vi "Read lockin vs time_1.0.vi"(8 "stop":bool, 10 "Comments":string="SA02610M 20130128\ncool down\n", 11 "folder name":string="monitor lockin") -> (1 "X1":cluster{"Y":dbl[], "Y":dbl[]}[](graph), 3 "Temp vs Time":cluster{"Y":dbl[], "Y":dbl[]}[](graph), 5 "X4":cluster{"Y":dbl[], "Y":dbl[]}[](graph))   [LabVIEW 2013]
uses:
  <userlib>/Levylab/PPMS VI/Lock-in Globles.vi
  <userlib>/Levylab/PPMS VI/SubVI/ITX_Global.vi
  cryogenic ltd/state machine/state machine/Cryogeni Global 1.vi
  <vilib>/Utility/file.llb/Write To Spreadsheet File (string).vi
panel:
  in  "Tab Control":T1(tab)
  in  "milliseconds to wait":u32=1000
  out "Connected":string="I-:4\nV2+:28\nI+:1\nV1+:2\nV-:3\nV2-:5\n"
  in  "Lockins":i32[](array[numeric])=[0, 1, 2, 3, 4, 5]
  out "Array X":dbl[](array[numeric])
  out "Array Y":dbl[](array[numeric])
  out "X0":cluster{"Y":dbl[], "Y":dbl[]}[](graph)
  out "X2":cluster{"Y":dbl[], "Y":dbl[]}[](graph)
  out "X3":cluster{"Y":dbl[], "Y":dbl[]}[](graph)
  out "X5":cluster{"Y":dbl[], "Y":dbl[]}[](graph)
  out "R":cluster{"Y":dbl[], "Y":dbl[]}[](graph)
  in  "V1":i32
  in  "Current":i32
  in  "V2":i32
  out "B vs Time":cluster{"Y":dbl[], "Y":dbl[]}[](graph)
  out "R vs T":cluster{"Y":dbl[], "Y":dbl[]}[](graph)
  # "0,1,2,3 ect."
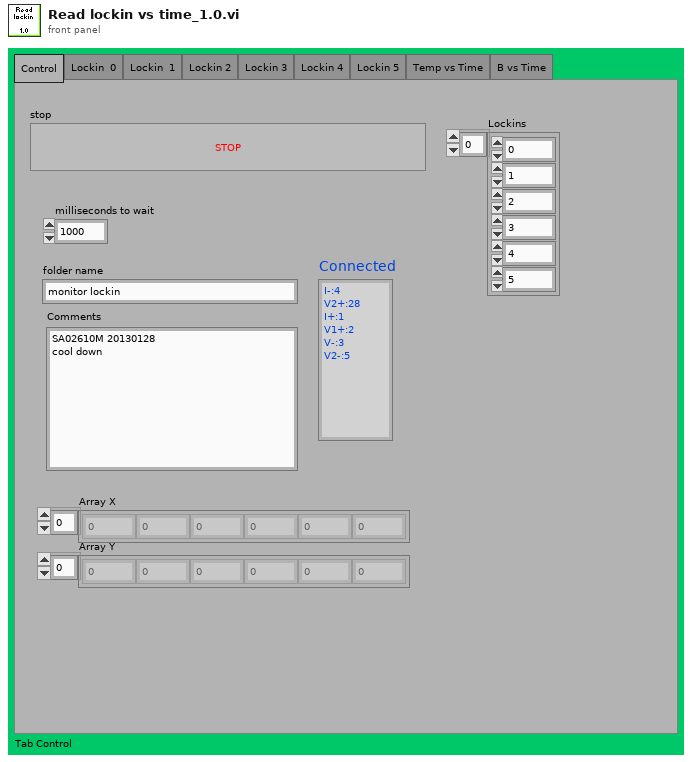
[diagram p1: front panel]
types:
  T1 = enum32{"Control", "Lockin  0", "Lockin  1", "Lockin 2", "Lockin 3", "Lockin 4", "Lockin 5", "Temp vs Time", "B vs Time"}
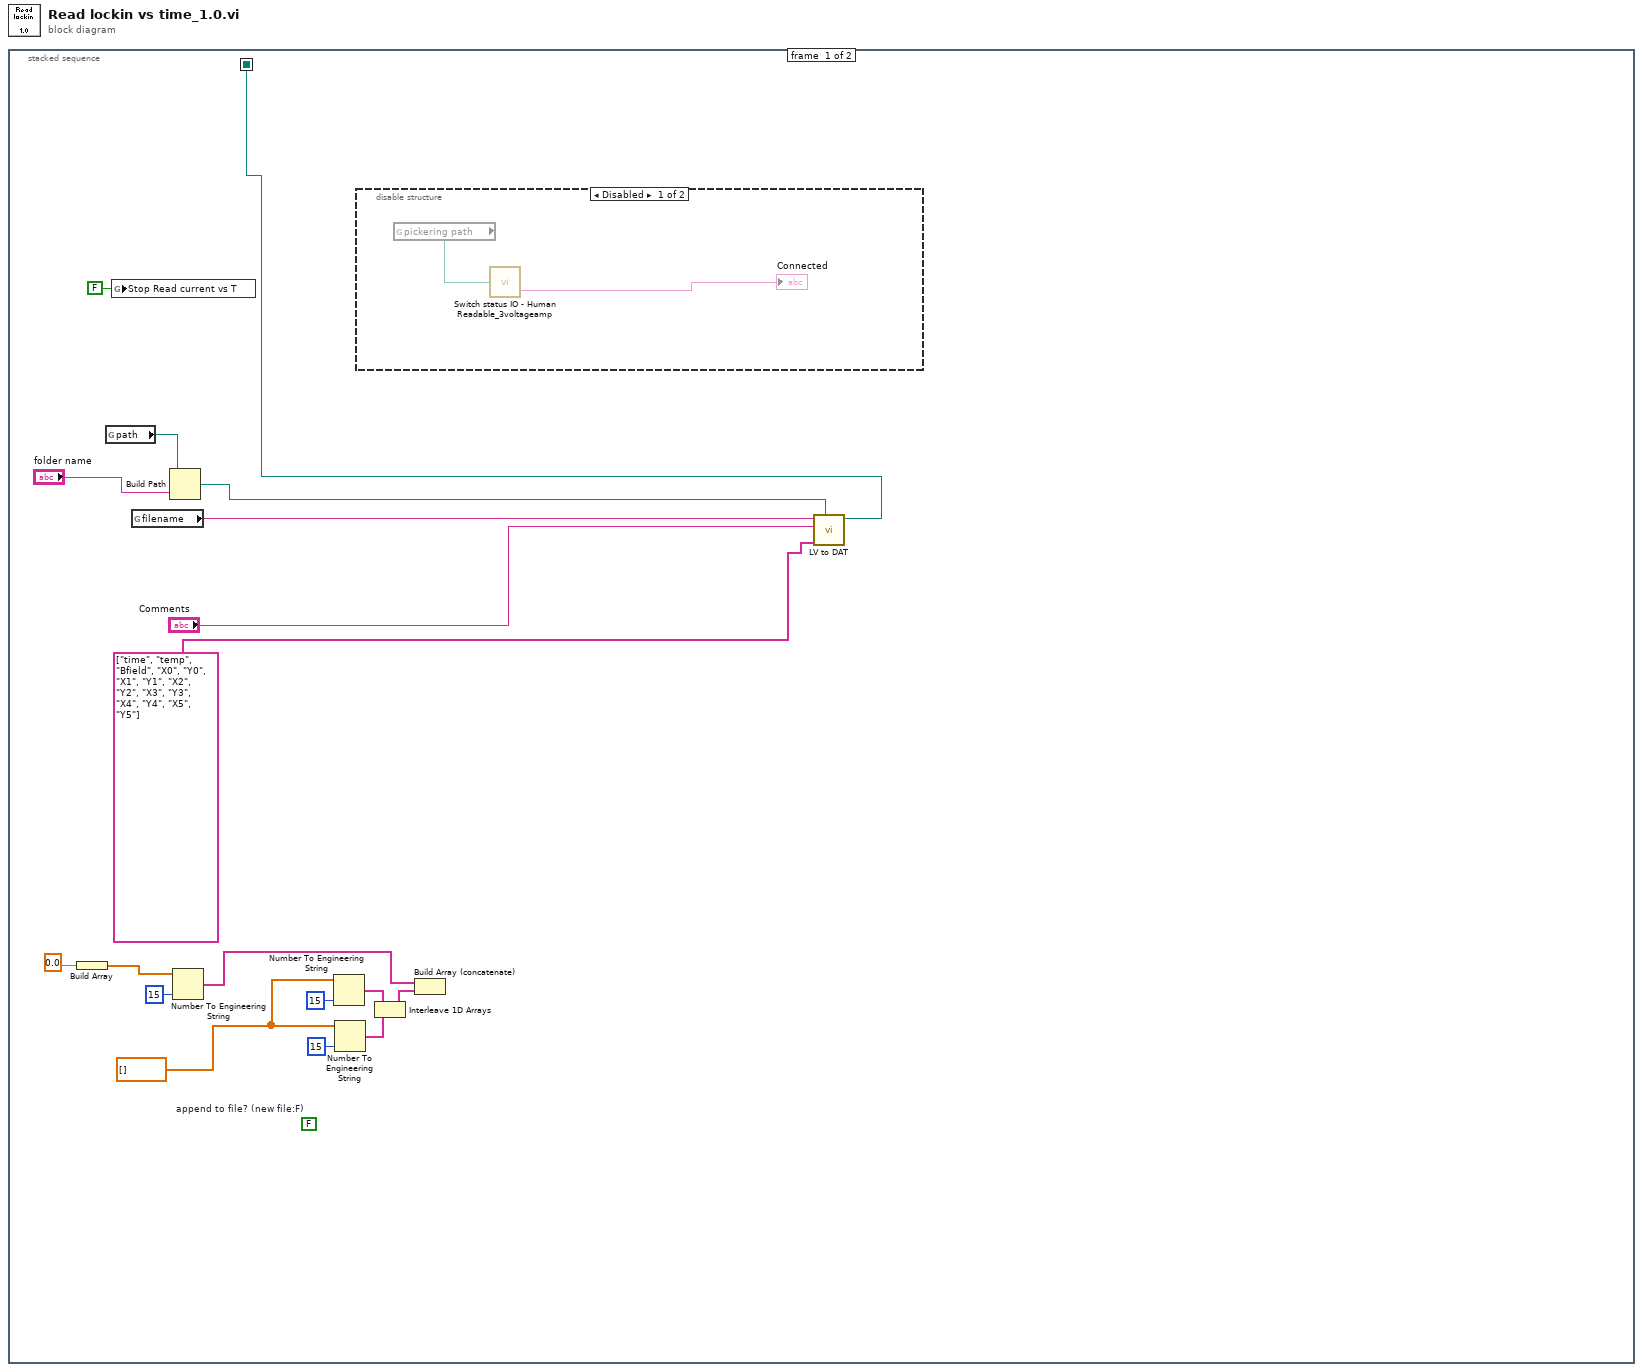
[diagram p0: block diagram]
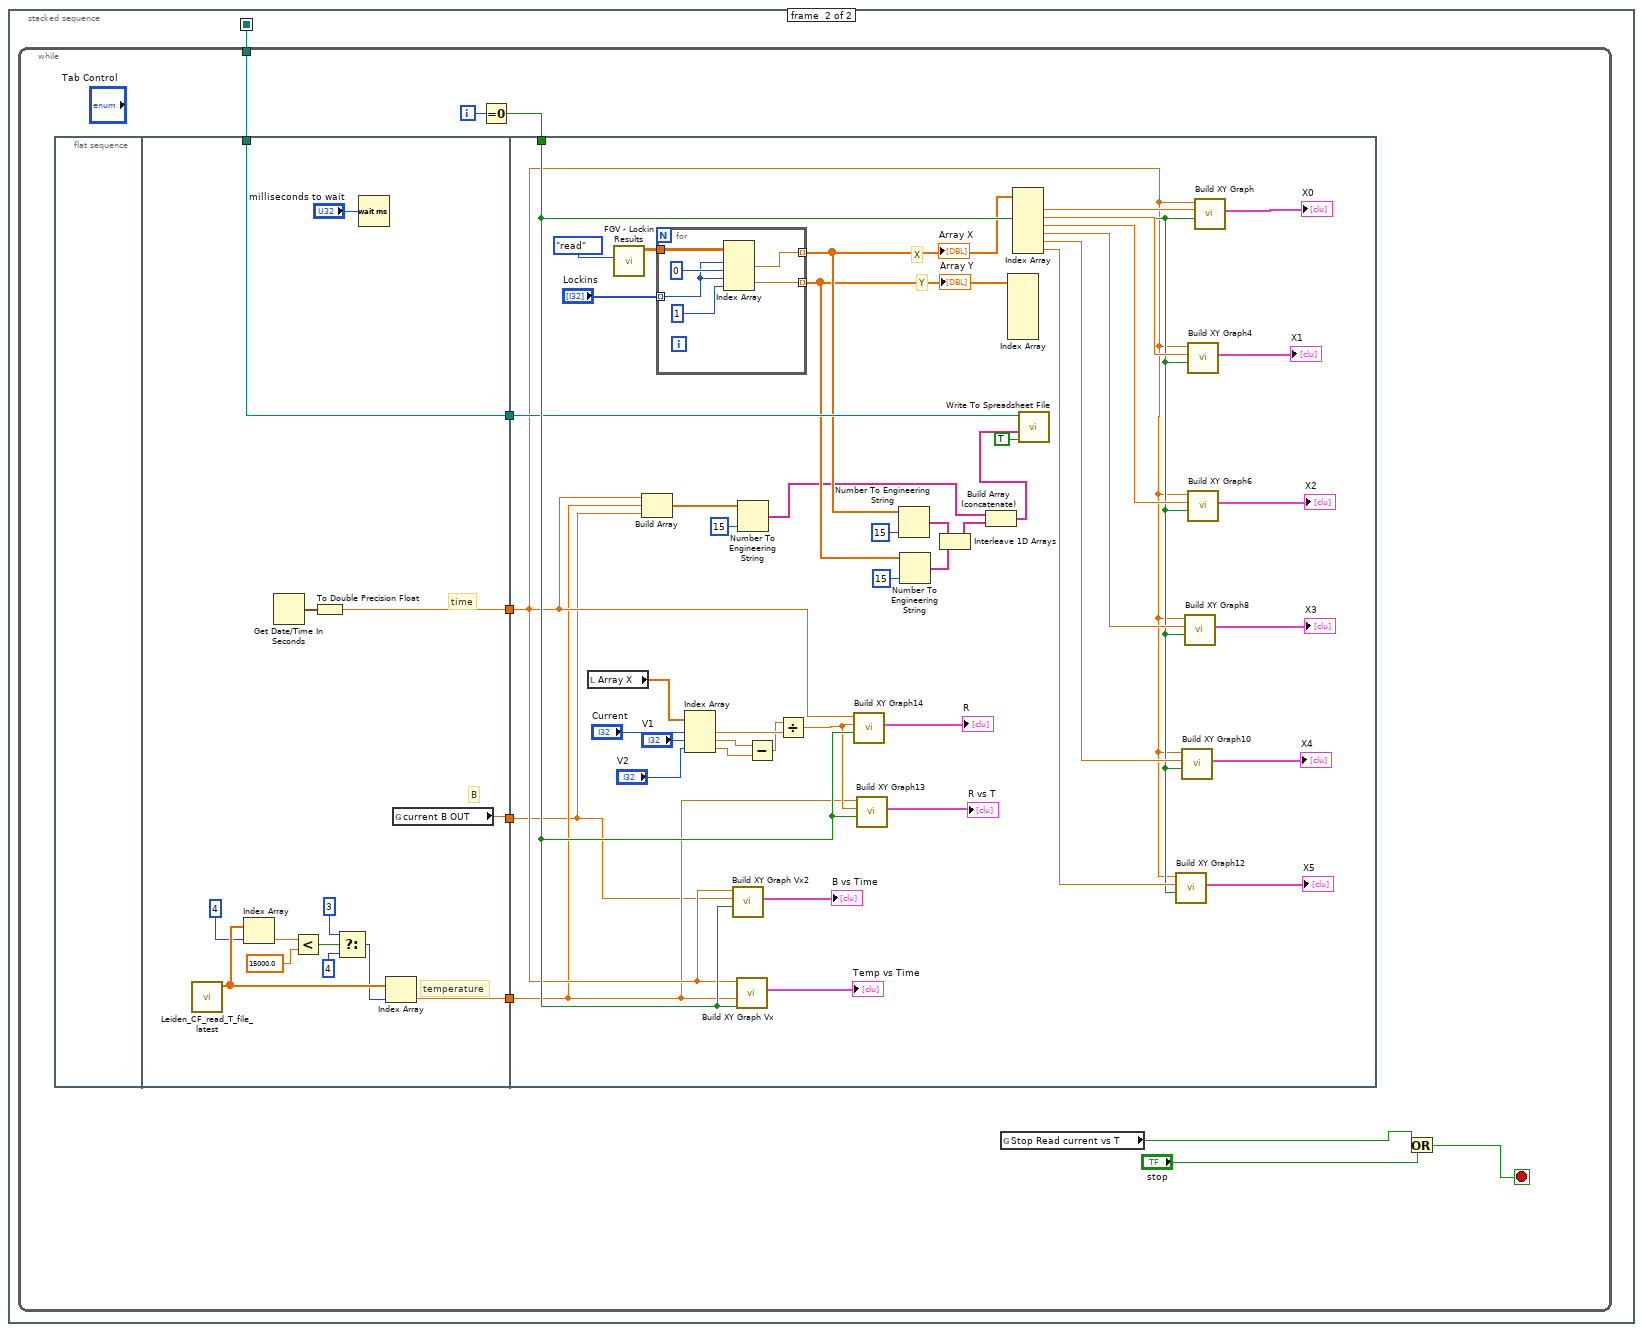
[diagram p3: hidden frame]
diagram:
  n1 = stacked-sequence {
    seq-local: [w1 _] -> [_ w23]
    frame #0 {
      w7 = dbl[] []
      w17 = FALSE  # append to file? (new file:F)
      n2 = Build Array(0.0) -> (w13:dbl[])
      n3 = global read "ITX_Global.vi" "path"() -> (w19:path)
      n4 = global write "Lock-in Globles.vi" "Stop Read current vs T"(FALSE ("Stop Read current vs T")) -> ()
      n5 = global read "ITX_Global.vi" "filename"() -> (w3:string)
      n6 = Build Path(base path=w19, name or relative path="folder name") -> (appended path=w2:path)
      n7 = Number To Engineering String(2:i16 15 ("precision (6)"), 4:w13) -> (0:w12:string[])  [unwired: 2 out]
      n8 = Number To Engineering String(2:i16 15 ("precision (6)"), 4:w7) -> (0:w11:string[])  [unwired: 2 out]
      n9 = Number To Engineering String(2:i16 15 ("precision (6)"), 4:w7) -> (0:w10:string[])  [unwired: 2 out]
      n10 = disable-structure shown="Disabled" {
        frame Disabled {
          n11 = global read "ITX_Global.vi" "pickering path"() -> (w21:path)
          n12 = call <userlib>:"Switch status IO - Human Readable_3voltageamp.vi"("Switch status"=w21) -> ("String"=→"Connected":string)  [unwired: 3 in]
        }
        frame Enabled {
        }
      }
      n13 = Interleave 1D Arrays(w11, w10) -> (w9:string[])
      n14 = Build Array (concatenate)(w12, w9) -> (w6:string[])
      n15 = call <userlib>:"LV to DAT.vi"("path"=w2, "wavenames (.Vx, etc)"=string[] ["time", "temp", "Bfield", "X0", "Y0", "X1", "Y1", "X2", "Y2", "X3", "Y3", "X4", "Y4", "X5", "Y5"], "Comments"="Comments", "filename"=w3) -> ("new file path (Not A Path if cancelled)"=w1:path)  [unwired: 7 in]
    }
    frame #1 {
      n16 = while {
        tunnel: w23 -> [w26]
        i -> [w33]
        stop <- w27 stop-if-true
        n17 = flat-sequence {
          tunnel: [w45] -> w31
          tunnel: [w44] -> w29
          tunnel: [w43] -> w28
          tunnel: w26 -> [w35]
          tunnel: [w35] -> w25
          tunnel: w32 -> [w69]
          tunnel: w31 -> [w57]
          tunnel: w29 -> [w56]
          tunnel: w28 -> [w55]
          tunnel: w25 -> [w67]
          frame #0 {
          }
          frame #1 {
            # "B"
            # "time"
            # "temperature"
            n18 = call "Leiden_CF_read_T_file_latest.vi"() -> ("T array"=w42:dbl[])  [unwired: 11 in]
            n19 = Index Array(array=w42, index=4) -> (element=w40:dbl)
            n20 = Get Date/Time In Seconds() -> (seconds since 1Jan1904=w46:timestamp)
            n21 = Less?(x=w40, y=15000.0) -> (x < y?=w38:bool)
            n22 = To Double Precision Float(number=w46) -> (double precision float=w45:dbl)
            n23 = Select(t=3 ("index"), s=w38, f=4 ("index")) -> (s? t:f=w34:i32)
            n24 = Wait (ms)(milliseconds to wait="milliseconds to wait") -> ()  [unwired: 1 out]
            n25 = Index Array(array=w42, index=w34) -> (element=w44:dbl)
            n26 = global read "Cryogeni Global 1.vi" "current B OUT"() -> (w43:dbl)
          }
          frame #2 {
            # "Y"
            # "X"
            n27 = local read "Array X"() -> (w64:dbl[])
            n28 = call <userlib>:"FGV - Lockin Results.vi"("Function"=enum16{"write", "read"}."read") -> ("Input Signals"=w70:dbl[][])  [unwired: 5 in, 1 out]
            n29 = Build Array(w57, w56, w55) -> (w54:dbl[])
            n30 = for {
              tunnel: w70 -> [w95]
              tunnel: "Lockins" -> [w96] mode=indexing
              tunnel: [w93] -> w61 mode=indexing
              tunnel: [w94] -> w59 mode=indexing
              n31 = Index Array(array=w95, index (row) #1=w96, index (col) #1=0 ("disabled index (col)"), index (row) #2=w96, index (col) #2=1 ("disabled index (col)")) -> (element #1=w93:dbl, element #2=w94:dbl)
            }
            "Array X" <- w61
            "Array Y" <- w59
            n32 = Index Array(array=w64, index #1="Current", index #2="V1", index #3="V2") -> (element #1=w74:dbl, element #2=w63:dbl, element #3=w62:dbl)
            n33 = call "Build XY Graph Vx2"("Reset"=w69, "Y Input"=w55, "X Input"=w57) -> ("XY Graph"=→"B vs Time":cluster{"Y":dbl[], "Y":dbl[]}[])  [unwired: 2 in, 6 out]
            n34 = call "Build XY Graph Vx"("Reset"=w69, "Y Input"=w56, "X Input"=w57) -> ("XY Graph"=→"Temp vs Time":cluster{"Y":dbl[], "Y":dbl[]}[])  [unwired: 2 in, 6 out]
            n35 = Number To Engineering String(2:i16 15 ("precision (6)"), 4:w54) -> (0:w53:string[])  [unwired: 2 out]
            n36 = Subtract(x=w63, y=w62) -> (x-y=w65:dbl)
            n37 = Divide(x=w65, y=w74) -> (x/y=w66:dbl)
            n38 = call "Build XY Graph14"("Reset"=w69, "Y Input"=w66, "X Input"=w57) -> ("XY Graph"=→"R":cluster{"Y":dbl[], "Y":dbl[]}[])  [unwired: 2 in, 6 out]
            n39 = call "Build XY Graph13"("Reset"=w69, "Y Input"=w66, "X Input"=w56) -> ("XY Graph"=→"R vs T":cluster{"Y":dbl[], "Y":dbl[]}[])  [unwired: 2 in, 6 out]
            n40 = Number To Engineering String(2:i16 15 ("precision (6)"), 4:w61) -> (0:w50:string[])  [unwired: 2 out]
            n41 = Number To Engineering String(2:i16 15 ("precision (6)"), 4:w59) -> (0:w49:string[])  [unwired: 2 out]
            n42 = Interleave 1D Arrays(w50, w49) -> (w48:string[])
            n43 = Build Array (concatenate)(w53, w48) -> (w52:string[])
            n44 = Index Array(array=w59) -> ()  [unwired: 6 in, 6 out]
            n45 = Index Array(array=w61) -> (element #1=w90:dbl, element #2=w88:dbl, element #3=w86:dbl, element #4=w84:dbl, element #5=w82:dbl, element #6=w80:dbl)  [unwired: 6 in]
            n46 = call-poly <vilib>:"Write To Spreadsheet File.vi"("append to file? (new file:F)"=TRUE, "1D data"=w52, "file path (dialog if empty)"=w67) -> ()  [unwired: 5 in, 1 out]
            n47 = call "Build XY Graph12"("Reset"=w69, "Y Input"=w80, "X Input"=w57) -> ("XY Graph"=→"X5":cluster{"Y":dbl[], "Y":dbl[]}[])  [unwired: 2 in, 6 out]
            n48 = call "Build XY Graph10"("Reset"=w69, "Y Input"=w82, "X Input"=w57) -> ("XY Graph"=→"X4":cluster{"Y":dbl[], "Y":dbl[]}[])  [unwired: 2 in, 6 out]
            n49 = call "Build XY Graph8"("Reset"=w69, "Y Input"=w84, "X Input"=w57) -> ("XY Graph"=→"X3":cluster{"Y":dbl[], "Y":dbl[]}[])  [unwired: 2 in, 6 out]
            n50 = call "Build XY Graph4"("Reset"=w69, "Y Input"=w88, "X Input"=w57) -> ("XY Graph"=→"X1":cluster{"Y":dbl[], "Y":dbl[]}[])  [unwired: 2 in, 6 out]
            n51 = call "Build XY Graph6"("Reset"=w69, "Y Input"=w86, "X Input"=w57) -> ("XY Graph"=→"X2":cluster{"Y":dbl[], "Y":dbl[]}[])  [unwired: 2 in, 6 out]
            n52 = call "Build XY Graph"("Reset"=w69, "Y Input"=w90, "X Input"=w57) -> ("XY Graph"=→"X0":cluster{"Y":dbl[], "Y":dbl[]}[])  [unwired: 2 in, 6 out]
          }
        }
        n53 = Equal To 0?(x=w33) -> (x = 0?=w32:bool)
        n54 = global read "Lock-in Globles.vi" "Stop Read current vs T"() -> (w24:bool)
        n55 = Or(x=w24, y="stop") -> (x .or. y?=w27:bool)
      }
    }
  }
